vi "test Verify with Regex Scrubber with Numbered Replacement.vi"(8 "error in":errorcluster, 11 "Test Case In":refnum<class "LUnit Extensions Tests.lvclass">) -> (0 "error out":errorcluster, 3 "Test Case Out":refnum<class "LUnit Extensions Tests.lvclass">)   [LabVIEW 2020, in "LUnit Extensions Tests.lvclass"]
uses:
  LUnit Extensions Tests.lvclass
  C:/Program Files/National Instruments/LabVIEW 2020/vi.lib/Astemes/LUnit/Test Case.lvclass
  Source/Approval Tests/Options.ctl
  Source/Approval Tests/Reporter/Reporter.lvclass
  Source/Approval Tests/Namer/Namer.lvclass
  Source/Approval Tests/Scrubber/Scrubber.lvclass
  Source/Approval Tests/Regex Scrubber Count Unique/Regex Scrubber Count Unique.lvclass
  C:/Users/SAS/Desktop/ApprovalTests.LabVIEW/Source/Approval Tests/Scrubber/Scrubber.lvclass
  Source/Approval Tests/Regex Scrubber Count Unique/Regex Scrubber Count Unique.lvclass/Regex Scrubber Count Unique.ctl
  <vilib>/Astemes/LUnit/Test Case.lvclass/Test Case.ctl
  240f995d-3744-484a-8956-6f48e6079b93.vi
  Source/Approval Tests/Regex Scrubber Count Unique/Write Regex.vi
  Source/Approval Tests/Regex Scrubber Count Unique/Write Prefix.vi
  240f995d-3744-484a-8956-6f48e6079b93.vi/1e051690-6811-4db0-8b8f-f6ad9423d026.vi
  <vilib>/Astemes/LUnit/Palette/Pass If.vi
  240f995d-3744-484a-8956-6f48e6079b93.vi/1e051690-6811-4db0-8b8f-f6ad9423d026.vi/93c5622b-9fb7-41e0-8c76-3fde37e94e34.vi
  <vilib>/Astemes/LUnit/Append Fail Result.vi
  <vilib>/Astemes/LUnit/Append Pass Result.vi
  Source/Approval Tests/Replace with Caller if Empty.vi
  Source/Approval Tests/conv EOL.vi
  <vilib>/Utility/libraryn.llb/Check if File or Folder Exists.vi
  LUnit Extensions Tests.lvclass/LUnit Extensions Tests.ctl
  Source/Approval Tests/Approval Tests.lvlib
  C:/Users/SAS/Desktop/ApprovalTests.LabVIEW/Source/Approval Tests/Regex Scrubber Count Unique/Regex Scrubber Count Unique.lvclass
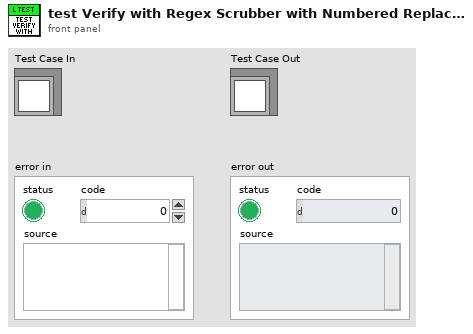
[diagram p1: front panel]
types:
  T1 = typedef "Approval Tests.lvlib/Options.ctl" = cluster{"Reporter":refnum<class "Reporter.lvclass">, "Extension(txt)":string, "Namer":refnum<class "Namer.lvclass">, "Scrubber":refnum<class "Scrubber.lvclass">, "Test Label":string}
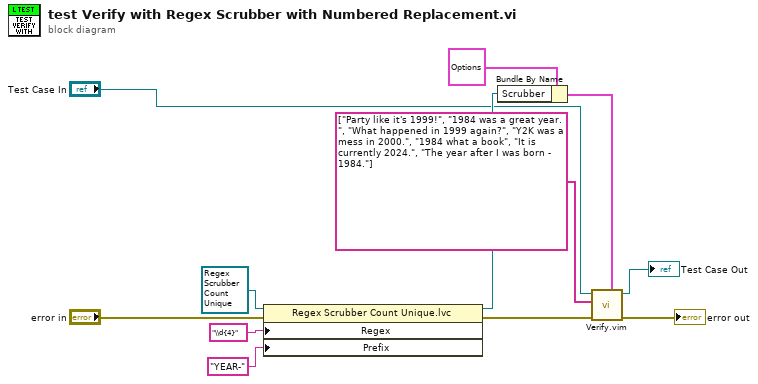
[diagram p0: block diagram]
diagram:
  n1 = property on="Property Node" class="Regex Scrubber Count Unique.lvc"(reference=refnum<class "Regex Scrubber Count Unique.lvclass"> refnum ("Approval Tests.lvlib:Regex Scrubber with Numbered Replacement.lvclass"), error in="error in", "Regex"="\\d{4}", "Prefix"="YEAR-" ("Replacement")) -> (reference out=w7:refnum<class "Regex Scrubber Count Unique.lvclass">, error out=w10:errorcluster)
  n2 = Bundle By Name(cluster=T1 {"Reporter"=refnum, "Extension(txt)"="", "Namer"=refnum, "Scrubber"=refnum, "Test Label"=""} ("Options"), "Scrubber"=w7) -> (w1:T1)
  n3 = call "Verify.vim"("Options"=w1, "error in"=w10, "Test Data"=string[] ["Party like it's 1999!", "1984 was a great year.", "What happened in 1999 again?", "Y2K was a mess in 2000.", "1984 what a book", "It is currently 2024.", "The year after I was born - 1984."], "LUnit Test Case In"="Test Case In") -> ("error out"=→"error out":errorcluster, "LUnit Test Case Out"=→"Test Case Out":refnum<class "LUnit Extensions Tests.lvclass">)  [unwired: 6 in]
